vi "DSF.Engine.Framework.Set Status.vi"(10 "Status":refnum<class "Framework Status.lvclass">, 11 "Framework in":refnum<class "DSF.Engine.Framework.lvclass">) -> (3 "Framework out":refnum<class "DSF.Engine.Framework.lvclass">)   [LabVIEW 2017, in "Data Sharing Framework Engine.lvlib" / "DSF.Engine.Framework.lvclass"]
uses:
  DSF.Engine.Framework.lvclass
  Source/Data Sharing Framework Core/Engine/Execution/Framework Status/Framework Status.lvclass
  DSF.Engine.Framework.lvclass/DSF.Engine.Framework.ctl
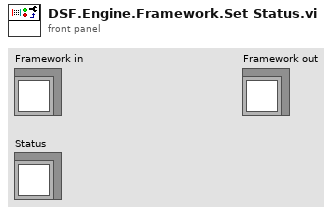
[diagram p1: front panel]
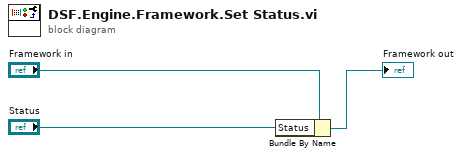
[diagram p0: block diagram]
diagram:
  n1 = Bundle By Name(cluster="Framework in", "Status"="Status") -> (→"Framework out":refnum<class "DSF.Engine.Framework.lvclass">)
